vi "Init Log.vi"(8 "error in (no error)":errorcluster, 11 "S4GUI in":refnum<class "S4GUI.lvclass">) -> (0 "error out":errorcluster, 3 "S4GUI out":refnum<class "S4GUI.lvclass">)   [LabVIEW 2018, in "S4GUI.lvclass"]
uses:
  S4GUI.lvclass
  S4GUI.lvclass/S4GUI.ctl
  Log/Log.lvclass
  Acquisition/Acquisition.lvclass
  Instrument/Instrument.lvclass
  TCS/TCS.lvclass
  SyncBox/Sync Box.lvclass
  TelFocus/TelFocus.lvclass
  Comm/Stream/Stream.lvclass
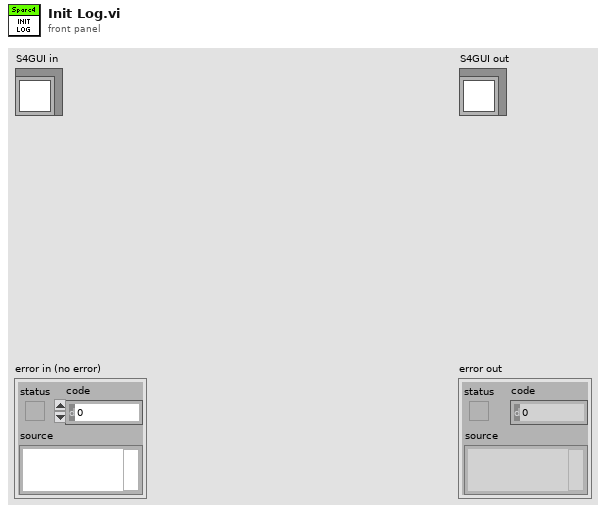
[diagram p1: front panel]
types:
  T1 = enum16{"open", "replace", "create", "open or create", "replace or create", "replace or create with confirmation"}
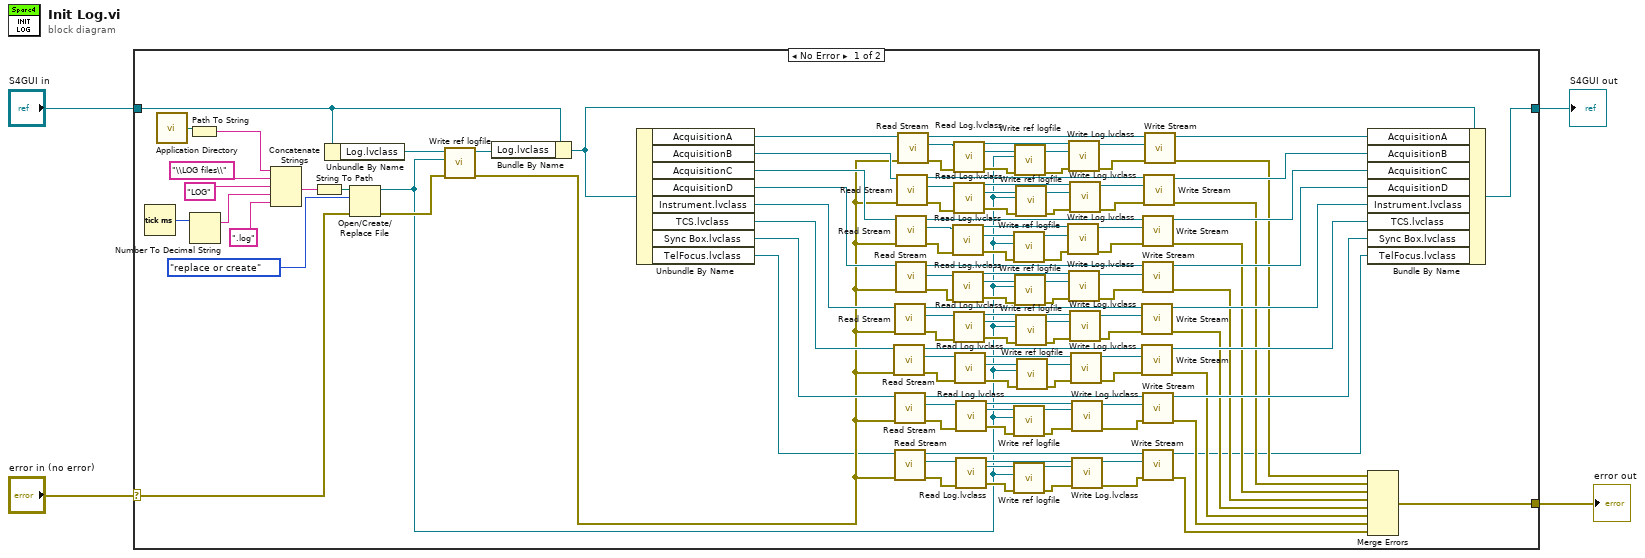
[diagram p0: block diagram]
diagram:
  n1 = case shown="No Error" "error in (no error)" {
    selector: "error in (no error)" -> [w124 w130]
    tunnel: [w99 w130] -> w3
    tunnel: [w121 w129] -> w1
    tunnel: "S4GUI in" -> [w25 w129]
    frame No Error {
      n2 = Tick Count (ms)() -> (millisecond timer value=w96:u32)
      n3 = call <vilib>:"Application Directory.vi"() -> ("Application Directory"=w127:path)
      n4 = Path To String(path=w127) -> (string=w21:string)
      n5 = Number To Decimal String(number=w96) -> (decimal integer string=w95:string)  [unwired: 1 in]
      n6 = Concatenate Strings(w21, "\\LOG files\\" ("string"), "LOG" ("string"), w95, ".log" ("string")) -> (w125:string)
      n7 = String To Path(string=w125) -> (path=w126:path)
      n8 = Unbundle By Name(w25) -> ("Log.lvclass"=w23:refnum<class "Log.lvclass">)
      n9 = Open/Create/Replace File(file path (use dialog)=w126, error in=w124, operation (0:open)=T1."replace or create") -> (refnum out=w5:refnum<file>, error out=w24:errorcluster)  [unwired: 3 in, 1 out]
      n10 = call-dynamic "Write ref logfile.vi"("error in (no error)"=w24, "ref logfile"=w5, "Log in"=w23) -> ("error out"=w12:errorcluster, "Log out"=w22:refnum<class "Log.lvclass">)  [unwired: 7 in]
      n11 = Bundle By Name(cluster=w25, "Log.lvclass"=w22) -> (w122:refnum<class "S4GUI.lvclass">)
      n12 = Unbundle By Name(w122) -> ("AcquisitionA"=w120:refnum<class "Acquisition.lvclass">, "AcquisitionB"=w119:refnum<class "Acquisition.lvclass">, "AcquisitionC"=w118:refnum<class "Acquisition.lvclass">, "AcquisitionD"=w117:refnum<class "Acquisition.lvclass">, "Instrument.lvclass"=w116:refnum<class "Instrument.lvclass">, "TCS.lvclass"=w115:refnum<class "TCS.lvclass">, "Sync Box.lvclass"=w114:refnum<class "Sync Box.lvclass">, "TelFocus.lvclass"=w11:refnum<class "TelFocus.lvclass">)
      n13 = call-dynamic "Read Stream.vi"("error in (no error)"=w12, "Server in"=w115) -> ("error out"=w31:errorcluster, "Stream.lvclass"=w32:refnum<class "Stream.lvclass">, "Server out"=w35:refnum<class "TCS.lvclass">)  [unwired: 7 in]
      n14 = call-dynamic "Read Stream.vi"("error in (no error)"=w12, "Server in"=w116) -> ("error out"=w47:errorcluster, "Stream.lvclass"=w49:refnum<class "Stream.lvclass">, "Server out"=w50:refnum<class "Instrument.lvclass">)  [unwired: 7 in]
      n15 = call-dynamic "Read Stream.vi"("error in (no error)"=w12, "Server in"=w114) -> ("error out"=w28:errorcluster, "Stream.lvclass"=w29:refnum<class "Stream.lvclass">, "Server out"=w30:refnum<class "Sync Box.lvclass">)  [unwired: 7 in]
      n16 = call-dynamic "Read Stream.vi"("error in (no error)"=w12, "Server in"=w11) -> ("error out"=w14:errorcluster, "Stream.lvclass"=w15:refnum<class "Stream.lvclass">, "Server out"=w10:refnum<class "TelFocus.lvclass">)  [unwired: 7 in]
      n17 = call-dynamic "Read Stream.vi"("error in (no error)"=w12, "Server in"=w118) -> ("error out"=w62:errorcluster, "Stream.lvclass"=w64:refnum<class "Stream.lvclass">, "Server out"=w65:refnum<class "Acquisition.lvclass">)  [unwired: 7 in]
      n18 = call-dynamic "Read Stream.vi"("error in (no error)"=w12, "Server in"=w117) -> ("error out"=w57:errorcluster, "Stream.lvclass"=w56:refnum<class "Stream.lvclass">, "Server out"=w60:refnum<class "Acquisition.lvclass">)  [unwired: 7 in]
      n19 = call-dynamic "Read Stream.vi"("error in (no error)"=w12, "Server in"=w119) -> ("error out"=w80:errorcluster, "Stream.lvclass"=w79:refnum<class "Stream.lvclass">, "Server out"=w77:refnum<class "Acquisition.lvclass">)  [unwired: 7 in]
      n20 = call-dynamic "Read Stream.vi"("error in (no error)"=w12, "Server in"=w120) -> ("error out"=w90:errorcluster, "Stream.lvclass"=w94:refnum<class "Stream.lvclass">, "Server out"=w123:refnum<class "Acquisition.lvclass">)  [unwired: 7 in]
      n21 = call-dynamic "Read Log.lvclass.vi"("error in (no error)"=w62, "Comm in"=w64) -> ("error out"=w72:errorcluster, "Log.lvclass"=w75:refnum<class "Log.lvclass">, "Comm out"=w74:refnum<class "Stream.lvclass">)  [unwired: 7 in]
      n22 = call-dynamic "Read Log.lvclass.vi"("error in (no error)"=w57, "Comm in"=w56) -> ("error out"=w67:errorcluster, "Log.lvclass"=w70:refnum<class "Log.lvclass">, "Comm out"=w69:refnum<class "Stream.lvclass">)  [unwired: 7 in]
      n23 = call-dynamic "Read Log.lvclass.vi"("error in (no error)"=w90, "Comm in"=w94) -> ("error out"=w89:errorcluster, "Log.lvclass"=w93:refnum<class "Log.lvclass">, "Comm out"=w92:refnum<class "Stream.lvclass">)  [unwired: 7 in]
      n24 = call-dynamic "Read Log.lvclass.vi"("error in (no error)"=w80, "Comm in"=w79) -> ("error out"=w82:errorcluster, "Log.lvclass"=w85:refnum<class "Log.lvclass">, "Comm out"=w84:refnum<class "Stream.lvclass">)  [unwired: 7 in]
      n25 = call-dynamic "Read Log.lvclass.vi"("error in (no error)"=w47, "Comm in"=w49) -> ("error out"=w52:errorcluster, "Log.lvclass"=w55:refnum<class "Log.lvclass">, "Comm out"=w54:refnum<class "Stream.lvclass">)  [unwired: 7 in]
      n26 = call-dynamic "Read Log.lvclass.vi"("error in (no error)"=w31, "Comm in"=w32) -> ("error out"=w42:errorcluster, "Log.lvclass"=w45:refnum<class "Log.lvclass">, "Comm out"=w44:refnum<class "Stream.lvclass">)  [unwired: 7 in]
      n27 = call-dynamic "Read Log.lvclass.vi"("error in (no error)"=w28, "Comm in"=w29) -> ("error out"=w37:errorcluster, "Log.lvclass"=w40:refnum<class "Log.lvclass">, "Comm out"=w39:refnum<class "Stream.lvclass">)  [unwired: 7 in]
      n28 = call-dynamic "Read Log.lvclass.vi"("error in (no error)"=w14, "Comm in"=w15) -> ("error out"=w17:errorcluster, "Log.lvclass"=w19:refnum<class "Log.lvclass">, "Comm out"=w8:refnum<class "Stream.lvclass">)  [unwired: 7 in]
      n29 = call-dynamic "Write ref logfile.vi"("error in (no error)"=w72, "ref logfile"=w5, "Log in"=w75) -> ("error out"=w71:errorcluster, "Log out"=w73:refnum<class "Log.lvclass">)  [unwired: 7 in]
      n30 = call-dynamic "Write ref logfile.vi"("error in (no error)"=w37, "ref logfile"=w5, "Log in"=w40) -> ("error out"=w36:errorcluster, "Log out"=w38:refnum<class "Log.lvclass">)  [unwired: 7 in]
      n31 = call-dynamic "Write ref logfile.vi"("error in (no error)"=w17, "ref logfile"=w5, "Log in"=w19) -> ("error out"=w16:errorcluster, "Log out"=w18:refnum<class "Log.lvclass">)  [unwired: 7 in]
      n32 = call-dynamic "Write ref logfile.vi"("error in (no error)"=w89, "ref logfile"=w5, "Log in"=w93) -> ("error out"=w88:errorcluster, "Log out"=w91:refnum<class "Log.lvclass">)  [unwired: 7 in]
      n33 = call-dynamic "Write ref logfile.vi"("error in (no error)"=w67, "ref logfile"=w5, "Log in"=w70) -> ("error out"=w66:errorcluster, "Log out"=w68:refnum<class "Log.lvclass">)  [unwired: 7 in]
      n34 = call-dynamic "Write ref logfile.vi"("error in (no error)"=w82, "ref logfile"=w5, "Log in"=w85) -> ("error out"=w81:errorcluster, "Log out"=w83:refnum<class "Log.lvclass">)  [unwired: 7 in]
      n35 = call-dynamic "Write ref logfile.vi"("error in (no error)"=w52, "ref logfile"=w5, "Log in"=w55) -> ("error out"=w51:errorcluster, "Log out"=w53:refnum<class "Log.lvclass">)  [unwired: 7 in]
      n36 = call-dynamic "Write ref logfile.vi"("error in (no error)"=w42, "ref logfile"=w5, "Log in"=w45) -> ("error out"=w41:errorcluster, "Log out"=w43:refnum<class "Log.lvclass">)  [unwired: 7 in]
      n37 = call-dynamic "Write Log.lvclass.vi"("error in (no error)"=w71, "Log.lvclass"=w73, "Comm in"=w74) -> ("error out"=w61:errorcluster, "Comm out"=w63:refnum<class "Stream.lvclass">)  [unwired: 7 in]
      n38 = call-dynamic "Write Log.lvclass.vi"("error in (no error)"=w88, "Log.lvclass"=w91, "Comm in"=w92) -> ("error out"=w87:errorcluster, "Comm out"=w86:refnum<class "Stream.lvclass">)  [unwired: 7 in]
      n39 = call-dynamic "Write Log.lvclass.vi"("error in (no error)"=w66, "Log.lvclass"=w68, "Comm in"=w69) -> ("error out"=w58:errorcluster, "Comm out"=w59:refnum<class "Stream.lvclass">)  [unwired: 7 in]
      n40 = call-dynamic "Write Log.lvclass.vi"("error in (no error)"=w81, "Log.lvclass"=w83, "Comm in"=w84) -> ("error out"=w76:errorcluster, "Comm out"=w78:refnum<class "Stream.lvclass">)  [unwired: 7 in]
      n41 = call-dynamic "Write Log.lvclass.vi"("error in (no error)"=w51, "Log.lvclass"=w53, "Comm in"=w54) -> ("error out"=w46:errorcluster, "Comm out"=w48:refnum<class "Stream.lvclass">)  [unwired: 7 in]
      n42 = call-dynamic "Write Log.lvclass.vi"("error in (no error)"=w41, "Log.lvclass"=w43, "Comm in"=w44) -> ("error out"=w33:errorcluster, "Comm out"=w34:refnum<class "Stream.lvclass">)  [unwired: 7 in]
      n43 = call-dynamic "Write Log.lvclass.vi"("error in (no error)"=w36, "Log.lvclass"=w38, "Comm in"=w39) -> ("error out"=w27:errorcluster, "Comm out"=w26:refnum<class "Stream.lvclass">)  [unwired: 7 in]
      n44 = call-dynamic "Write Log.lvclass.vi"("error in (no error)"=w16, "Log.lvclass"=w18, "Comm in"=w8) -> ("error out"=w13:errorcluster, "Comm out"=w7:refnum<class "Stream.lvclass">)  [unwired: 7 in]
      n45 = call-dynamic "Write Stream.vi"("error in (no error)"=w46, "Stream.lvclass"=w48, "Server in"=w50) -> ("error out"=w102:errorcluster, "Server out"=w109:refnum<class "Instrument.lvclass">)  [unwired: 7 in]
      n46 = call-dynamic "Write Stream.vi"("error in (no error)"=w33, "Stream.lvclass"=w34, "Server in"=w35) -> ("error out"=w101:errorcluster, "Server out"=w108:refnum<class "TCS.lvclass">)  [unwired: 7 in]
      n47 = call-dynamic "Write Stream.vi"("error in (no error)"=w61, "Stream.lvclass"=w63, "Server in"=w65) -> ("error out"=w104:errorcluster, "Server out"=w111:refnum<class "Acquisition.lvclass">)  [unwired: 7 in]
      n48 = call-dynamic "Write Stream.vi"("error in (no error)"=w58, "Stream.lvclass"=w59, "Server in"=w60) -> ("error out"=w103:errorcluster, "Server out"=w110:refnum<class "Acquisition.lvclass">)  [unwired: 7 in]
      n49 = call-dynamic "Write Stream.vi"("error in (no error)"=w27, "Stream.lvclass"=w26, "Server in"=w30) -> ("error out"=w100:errorcluster, "Server out"=w107:refnum<class "Sync Box.lvclass">)  [unwired: 7 in]
      n50 = call-dynamic "Write Stream.vi"("error in (no error)"=w13, "Stream.lvclass"=w7, "Server in"=w10) -> ("error out"=w6:errorcluster, "Server out"=w9:refnum<class "TelFocus.lvclass">)  [unwired: 7 in]
      n51 = call-dynamic "Write Stream.vi"("error in (no error)"=w76, "Stream.lvclass"=w78, "Server in"=w77) -> ("error out"=w105:errorcluster, "Server out"=w112:refnum<class "Acquisition.lvclass">)  [unwired: 7 in]
      n52 = call-dynamic "Write Stream.vi"("error in (no error)"=w87, "Stream.lvclass"=w86, "Server in"=w123) -> ("error out"=w106:errorcluster, "Server out"=w113:refnum<class "Acquisition.lvclass">)  [unwired: 7 in]
      n53 = Bundle By Name(cluster=w122, "AcquisitionA"=w113, "AcquisitionB"=w112, "AcquisitionC"=w111, "AcquisitionD"=w110, "Instrument.lvclass"=w109, "TCS.lvclass"=w108, "Sync Box.lvclass"=w107, "TelFocus.lvclass"=w9) -> (w121:refnum<class "S4GUI.lvclass">)
      n54 = Merge Errors(w106, w105, w104, w103, w102, w101, w100, w6) -> (w99:errorcluster)
    }
    frame Error {
    }
  }
  "error out" <- w3
  "S4GUI out" <- w1
